vi "Periodic Tasks.vi"(8 "error in":errorcluster) -> ()   [LabVIEW 2016]
doc: "This VI runs in parallel to other tasks. It can contain as many user-defined periodic loops as you need. These can carry out PID or other sorts of timed response."
uses:
  <vilib>/Rock Robotics/WPI/DriverStation/WPI_DriverStationRobotMode2.ctl
  <vilib>/Rock Robotics/WPI/Utilities/WPI_GetSetVariantRefNum.vi
  Robot Global Data.vi
  <vilib>/Rock Robotics/WPI/RobotDrive/WPI_RobotDriveArcadeDrive_Standard(NoSaturation).vi
  <vilib>/Rock Robotics/Network Tables/NT Read String.vi
  <vilib>/Rock Robotics/Network Tables/NT Read Number.vi
  Drive Base Class/DriveBase.lvclass
panel:
  in  "Angle PID gains":T1
  out "Robot Mode":T2
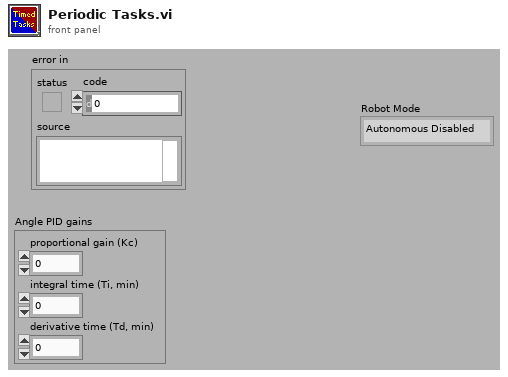
[diagram p1: front panel]
types:
  T1 = cluster{"proportional gain (Kc)":dbl, "integral time (Ti, min)":dbl, "derivative time (Td, min)":dbl}
  T2 = typedef "WPI_DriverStationRobotMode2.ctl" = enum16{"Autonomous Disabled", "Autonomous Enabled", "Teleop Disabled", "Teleop Enabled", "Disconnected", "Finish", "Test Disabled", "Test Enabled", "Emergency Stopped"}
  T3 = typedef "WPI_GyroDevRef.ctl" = cluster{"DevStatus":errorcluster, "Analog Channel":T4, "Offset":dbl, "Gain (VoltsPerDegree/Second)":dbl, "Gyro Type":enum16{"Analog", "XRS450"}, "Handle":i32, "SPI Bus":T5, "Device Found":bool, "Sample Rate":dbl, "Calibrate On Open":bool}
  T4 = typedef "FPGA_AIChannel.ctl" = enum8{"AI 0", "AI 1", "AI 2", "AI 3", "AI MXP 0", "AI MXP 1", "AI MXP 2", "AI MXP 3", "Invalid"}
  T5 = typedef "spi_bus.ctl" = enum16{"SPI On-Board, CS0", "SPI On-Board, CS1", "SPI On-Board, CS2", "SPI On-Board, CS3", "SPI MXP", "Invalid"}
  T6 = typedef "WPI_PotentiometerDevRef.ctl" = cluster{"DevStatus":errorcluster, "Analog Channel":T4, "Invert Output":bool}
  T7 = typedef "WPI_EncoderDevRef.ctl" = cluster{"DevStatus":errorcluster, "EncoderIndex":T8, "CounterIndex":T9, "DistancePerCount":dbl, "Decoding Type":T10}
  T8 = typedef "FPGA_EncoderIdx.ctl" = enum8{"Enc 0", "Enc 1", "Enc 2", "Enc 3", "Enc 4", "Enc 5", "Enc 6", "Enc 7", "Invalid"}
  T9 = typedef "FPGA_CounterCtrSystemIndex.ctl" = enum8{"Ctr 0", "Ctr 1", "Ctr 2", "Ctr 3", "Ctr 4", "Ctr 5", "Ctr 6", "Ctr 7", "Invalid"}
  T10 = typedef "WPI_EncoderType.ctl" = enum16{"1x", "2x", "4x"}
  T11 = cluster{"Right Encoder Distance":dbl, "Left Encoder Distance":dbl, "Right Encoder Velocity":dbl, "Left Encoder Velocity":dbl}
  T12 = cluster{"Yaw":dbl, "Roll":dbl, "Pitch":dbl, "Heading":dbl, "Fused Heading":dbl}
  T13 = typedef "WPI_RobotDriveDevRef.ctl" = cluster{"DevStatus":errorcluster, "Motors[]":T14[], "Square Inputs":bool, "Max Output":dbl}
  T14 = typedef "WPI_MotorControlDeviceRef.ctl" = cluster{"DeviceStatus":errorcluster, "Type":T15, "PWM":cluster{"PWM Channel":T16, "DeadBand":T17}, "CAN":cluster{"Device Number":u8, "SetOutput VI Ref":variant, "GetOutput VI Ref":variant, "Enable VI Ref":variant, "Disable VI Ref":variant, "Data":variant}, "Invert":bool}
  T15 = typedef "WPI_MotorControlType.ctl" = enum16{"PWM", "CAN"}
  T16 = typedef "FPGA_DIOPWMChannel.ctl" = enum8{"PWM 0", "PWM 1", "PWM 2", "PWM 3", "PWM 4", "PWM 5", "PWM 6", "PWM 7", "PWM 8", "PWM 9", "PWM MXP 0", "PWM MXP 1", "PWM MXP 2", "PWM MXP 3", "PWM MXP 4", "PWM MXP 5", "PWM MXP 6", "PWM MXP 7", "PWM MXP 8", "PWM MXP 9", "Invalid"}
  T17 = typedef "WPI_PWMDeadband.ctl" = cluster{"Name":string, "maxPositivePwm":i32, "minPositivePwm":i32, "centerPwm":i32, "maxNegativePwm":i32, "minNegativePwm":i32, "angularRange":u16}
  T18 = typedef "DriveBase.lvclass/DriveStates.ctl" = enum16{"Tank", "Arcade", "DriveStraight"}
  T19 = enum16{"open", "replace", "create", "open or create", "replace or create", "replace or create with confirmation"}
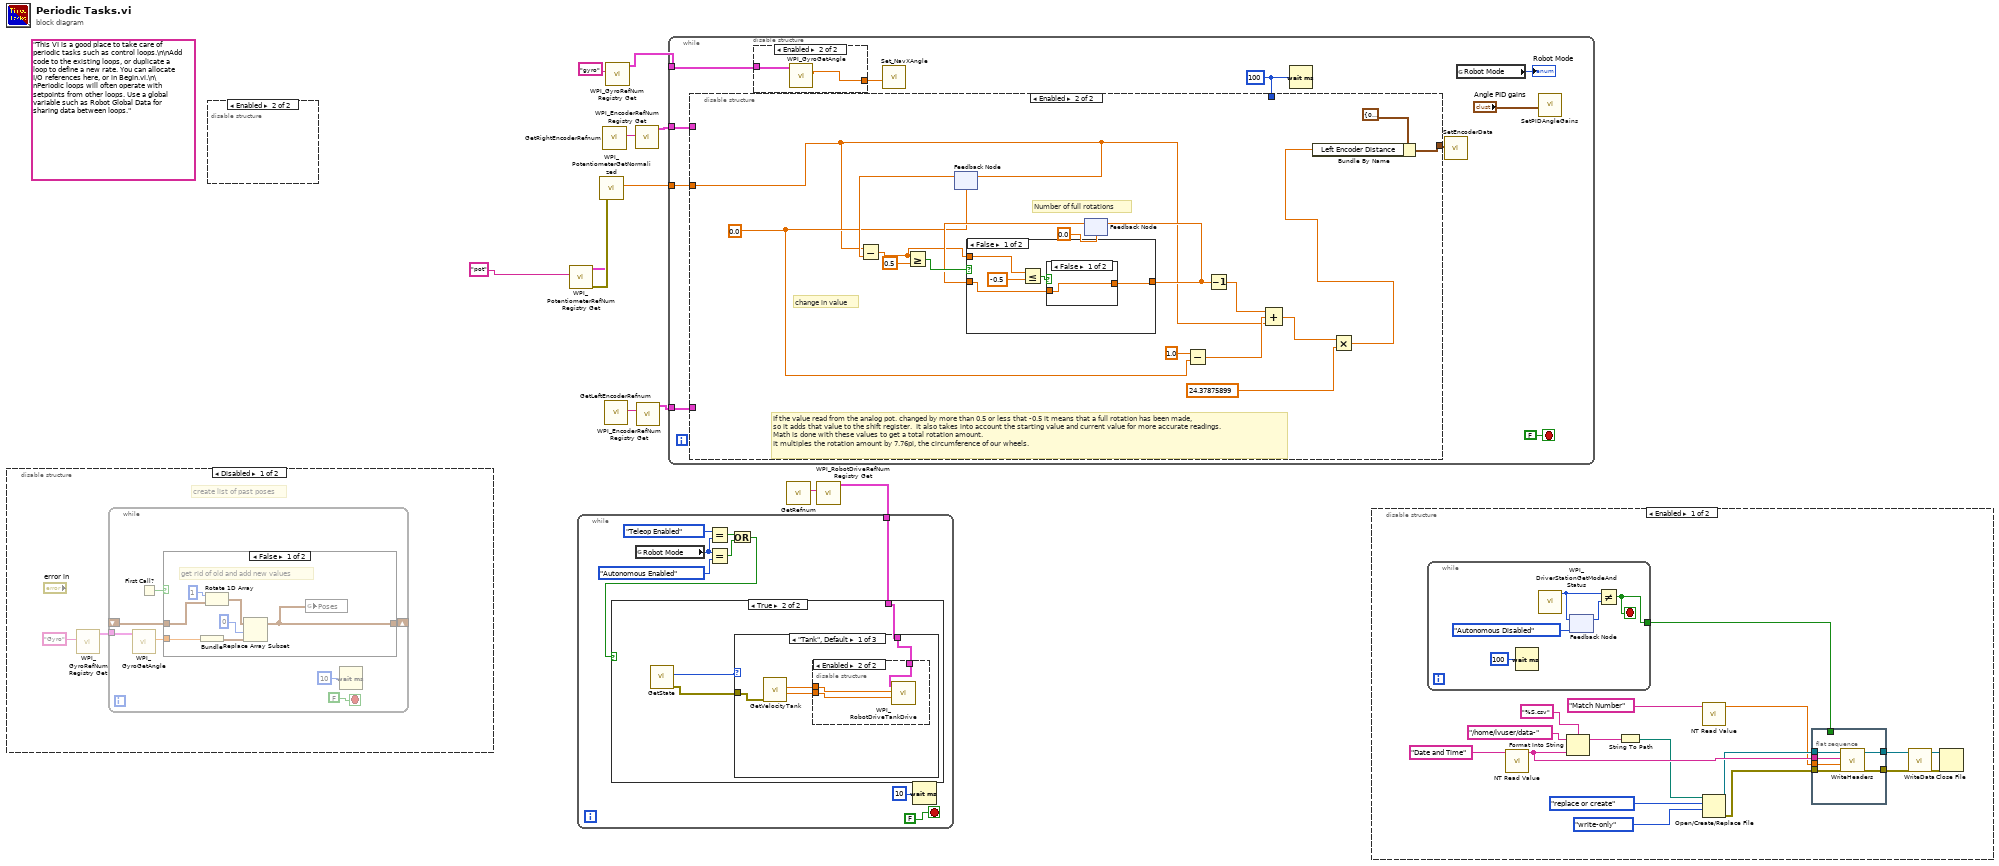
[diagram p0: block diagram]
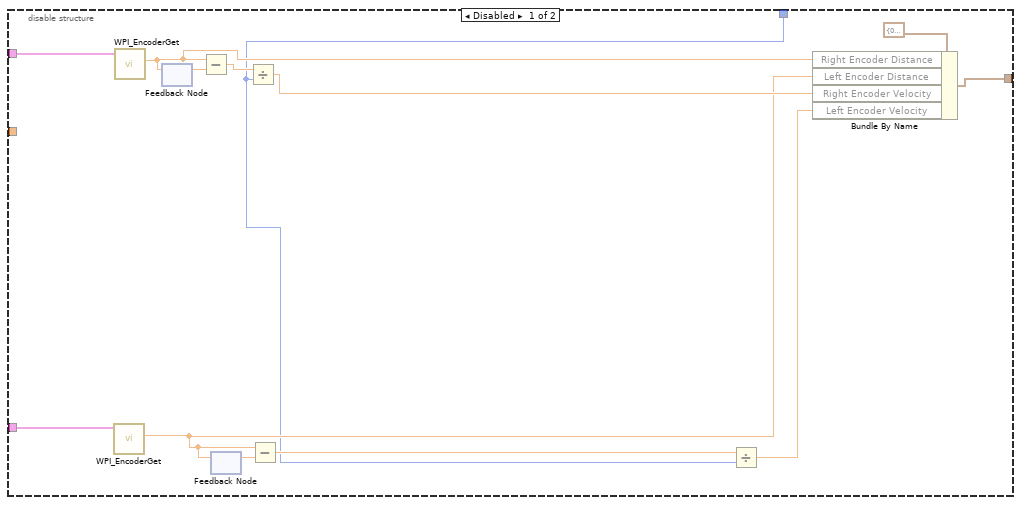
[diagram p2: hidden frame]
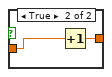
[diagram p3: hidden frame]
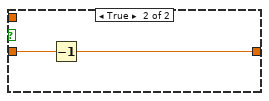
[diagram p4: hidden frame]
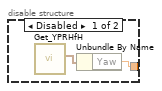
[diagram p5: hidden frame]
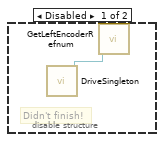
[diagram p7: hidden frame]
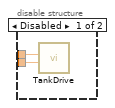
[diagram p9: hidden frame]
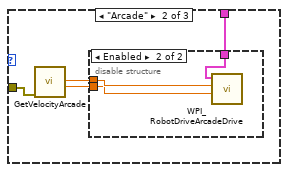
[diagram p10: hidden frame]
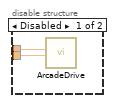
[diagram p11: hidden frame]
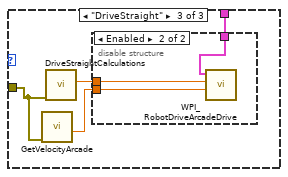
[diagram p12: hidden frame]
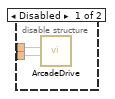
[diagram p13: hidden frame]
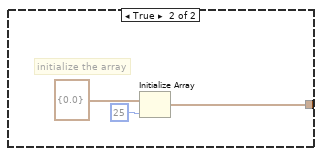
[diagram p14: hidden frame]
diagram:
  (unwired) "This VI is a good place to take care of periodic tasks such as control loops.\n\nAdd code to the existing loops, or duplicate a loop to define a new rate. You can allocate I/O references here, or in Begin.vi.\n\nPeriodic loops will often operate with setpoints from other loops. Use a global variable such as Robot Global Data for sharing data between loops."
  n1 = disable-structure shown="Disabled" {
    frame Disabled {
      # "create list of past poses"
      n2 = call <vilib>:"WPI_GyroRefNum Registry Get.vi"("refnum name"="Gyro") -> ("GyroDevRef"=w13:T3)  [unwired: 9 in, 1 out]
      n3 = while {
        tunnel: w13 -> [w19]
        shift-right: [w17] -> _
        shift-left: _ -> [w16]
        stop <- FALSE stop-if-true
        n4 = call <vilib>:"WPI_GyroGetAngle.vi"("GyroDevRef"=w19) -> ("Angle"=w15:dbl)  [unwired: 6 in, 4 out]
        n5 = First Call?() -> (First Call?: T/F=w18:bool)
        n6 = case shown="False" w18 {
          tunnel: [w22 w30] -> w17
          tunnel: w16 -> [w28 _]
          tunnel: w15 -> [w24 _]
          frame False {
            # "get rid of old and add new values"
            n7 = Bundle("Angle"=w24) -> (w23:cluster{"Angle":dbl})  [unwired: 1 in]
            n8 = Rotate 1D Array(1:w28, 2:1 ("n")) -> (0:w26:cluster{"theta":dbl}[])
            n9 = Replace Array Subset(array=w26, new element=w23, index=0) -> (w22:cluster{"theta":dbl}[])
            n10 = global write "Robot Global Data.vi" "Poses"(w22) -> ()
          }
          frame True {
            # "initialize the array"
            n11 = Initialize Array(cluster{"theta":dbl} {"theta"=0.0}, 25 ("dimension size")) -> (w30:cluster{"theta":dbl}[])
          }
        }
        n12 = Wait (ms)(milliseconds to wait=u32 10) -> ()  [unwired: 1 out]
      }
    }
    frame Enabled {
    }
  }
  n13 = disable-structure shown="Enabled" {
    frame Disabled {
      # "Didn't finish!"
      n14 = call "DriveSingleton.vi"() -> ("DriveBase.lvclass 2"=w32:refnum<class "DriveBase.lvclass">)  [unwired: 10 in, 1 out]
      n15 = call "GetLeftEncoderRefnum.vi"(11:w32) -> ()  [unwired: 10 in, 1 out]
    }
    frame Enabled {
    }
  }
  n16 = call <vilib>:"WPI_PotentiometerRefNum Registry Get.vi"("refnum name"="pot") -> ("error out"=w3:errorcluster, "PotDevRef"=w2:T6)  [unwired: 9 in]
  n17 = call <vilib>:"WPI_PotentiometerGetNormalized.vi"("error in"=w3, "PotDevRef"=w2) -> ("Normalized Value"=w4:dbl)  [unwired: 7 in, 2 out]
  n18 = call "GetRightEncoderRefnum.vi"() -> ("RightEncoderRefnum"=w5:string)  [unwired: 11 in]
  n19 = call "GetLeftEncoderRefnum.vi"() -> ("LeftEncoderRefnum"=w6:string)  [unwired: 11 in]
  n20 = call <vilib>:"WPI_GyroRefNum Registry Get.vi"("refnum name"="gyro") -> ("GyroDevRef"=w9:T3)  [unwired: 9 in, 1 out]
  n21 = call <vilib>:"WPI_EncoderRefNum Registry Get.vi"("refnum name"=w5) -> ("EncoderDevRef"=w8:T7)  [unwired: 9 in, 1 out]
  n22 = call <vilib>:"WPI_EncoderRefNum Registry Get.vi"("refnum name"=w6) -> ("EncoderDevRef"=w7:T7)  [unwired: 9 in, 1 out]
  n23 = while {
    tunnel: w9 -> [w38]
    tunnel: w8 -> [w37]
    tunnel: w7 -> [w36]
    tunnel: w4 -> [w33]
    stop <- FALSE stop-if-true
    w34 = u32 100 ("milliseconds to wait")
    n24 = disable-structure shown="Enabled" {
      disable-tunnel: w37 -> [w55 _]
      disable-tunnel: w36 -> [w54 _]
      disable-tunnel: [w44 w58] -> w35
      disable-tunnel: w34 -> [w43 _]
      disable-tunnel: w33 -> [_ w60]
      frame Disabled {
        n25 = call <vilib>:"WPI_EncoderGet.vi"("EncoderDevRef"=w54) -> ("Distance"=w46:dbl)  [unwired: 5 in, 5 out]
        n26 = call <vilib>:"WPI_EncoderGet.vi"("EncoderDevRef"=w55) -> ("Distance"=w52:dbl)  [unwired: 5 in, 5 out]
        n27 = feedback #1() -> (w53:dbl)  [unwired: 1 in]
        n28 = feedback-in #1(w52) -> ()
        n29 = Subtract(x=w52, y=w53) -> (x-y=w50:dbl)
        n30 = feedback #2() -> (w48:dbl)  [unwired: 1 in]
        n31 = feedback-in #2(w46) -> ()
        n32 = Divide(x=w50, y=w43) -> (x/y=w49:dbl)
        n33 = Subtract(x=w46, y=w48) -> (x-y=w47:dbl)
        n34 = Divide(x=w47, y=w43) -> (x/y=w45:dbl)
        n35 = Bundle By Name(cluster=T11 {"Right Encoder Distance"=0.0, "Left Encoder Distance"=0.0, "Right Encoder Velocity"=0.0, "Left Encoder Velocity"=0.0} ("Encoder Data"), "Right Encoder Distance"=w52, "Left Encoder Distance"=w46, "Right Encoder Velocity"=w49, "Left Encoder Velocity"=w45) -> (w44:T11)
      }
      frame Enabled {
        w61 = 0.0 ("y")
        # "change in value"
        # "Number of full rotations"
        # "If the value read from the analog pot. changed by more than 0.5 or less that -0.5 it means that a full rotation has been made, \nso it adds that value to the shift register.  It also takes into account the starting value and current value for more accurate readings.\nMath is done with these values to get a total rotation amount.\nIt multiples the rotation amount by 7.76pi, the circumference of our wheels."
        n36 = feedback #3(w61) -> (w64:dbl)
        n37 = Subtract(x=w60, y=w64) -> (x-y=w69:dbl)
        n38 = Greater Or Equal?(x=w69, y=0.5) -> (x >= y?=w71:bool)
        n39 = feedback-in #3(w60) -> ()
        n40 = feedback #4(0.0) -> (w70:dbl)
        n41 = case shown="False" w71 {
          tunnel: [w73 w82] -> w67
          tunnel: w70 -> [w74 w81]
          tunnel: w69 -> [w77 _]
          frame False {
            n42 = Less Or Equal?(x=w77, y=-0.5) -> (x <= y?=w75:bool)
            n43 = case shown="False" w75 {
              tunnel: w74 -> [w78 w80]
              tunnel: [w78 w79] -> w73
              frame False {
              }
              frame True {
                n44 = Increment(x=w80) -> (x+1=w79:dbl)
              }
            }
          }
          frame True {
            n45 = Decrement(x=w81) -> (x-1=w82:dbl)
          }
        }
        n46 = feedback-in #4(w67) -> ()
        n47 = Subtract(x=1.0, y=w61) -> (x-y=w65:dbl)
        n48 = Decrement(x=w67) -> (x-1=w66:dbl)
        n49 = Compound Arithmetic op=ADD(w66, w65, w60) -> (w62:dbl)
        n50 = Multiply(x=w62, y=24.37875899) -> (x*y=w57:dbl)
        n51 = Bundle By Name(cluster=T11 {"Right Encoder Distance"=0.0, "Left Encoder Distance"=0.0, "Right Encoder Velocity"=0.0, "Left Encoder Velocity"=0.0} ("Encoder Data"), "Left Encoder Distance"=w57) -> (w58:T11)
      }
    }
    n52 = disable-structure shown="Enabled" {
      disable-tunnel: [w83 w85] -> w42
      disable-tunnel: w38 -> [_ w86]
      frame Disabled {
        n53 = call <userlib>:"Get_YPRHfH.vi"() -> ("YRPHfH"=w84:T12)  [unwired: 11 in]
        n54 = Unbundle By Name(w84) -> ("Yaw"=w83:dbl)
      }
      frame Enabled {
        n55 = call <vilib>:"WPI_GyroGetAngle.vi"("GyroDevRef"=w86) -> ("Angle"=w85:dbl)  [unwired: 6 in, 4 out]
      }
    }
    n56 = call "Set_NavXAngle.vi"("NavX Angle"=w42) -> ()  [unwired: 11 in]
    n57 = Wait (ms)(milliseconds to wait=w34) -> ()  [unwired: 1 out]
    n58 = call "SetEncoderData.vi"("Encoder Data"=w35) -> ()  [unwired: 10 in, 1 out]
    n59 = global read "Robot Global Data.vi" "Robot Mode"() -> (→"Robot Mode":T2)
    n60 = call "SetPIDAngleGains.vi"("Angle PID gains"="Angle PID gains") -> ()  [unwired: 10 in, 1 out]
  }
  n61 = call "GetRefnum.vi"() -> ("RobotDriveRefnum"=w12:string)  [unwired: 10 in, 1 out]
  n62 = call <vilib>:"WPI_RobotDriveRefNum Registry Get.vi"("refnum name"=w12) -> ("RobotDriveDevRef"=w11:T13)  [unwired: 9 in, 1 out]
  n63 = while {
    tunnel: w11 -> [w93]
    stop <- FALSE stop-if-true
    n64 = global read "Robot Global Data.vi" "Robot Mode"() -> (w88:T2)
    n65 = Equal?(x=WPI_DriverStationRobotMode2."Teleop Enabled" ("Robot Mode"), y=w88) -> (x = y?=w91:bool)
    n66 = Equal?(x=w88, y=WPI_DriverStationRobotMode2."Autonomous Enabled" ("Robot Mode")) -> (x = y?=w90:bool)
    n67 = Or(x=w91, y=w90) -> (x .or. y?=w87:bool)
    n68 = case shown="True" w87 {
      tunnel: w93 -> [_ w98]
      frame False {
      }
      frame True {
        n69 = call "GetState.vi"() -> ("error out"=w96:errorcluster, "State"=w97:T18)  [unwired: 10 in]
        n70 = case shown="\"Tank\", Default" w97 {
          tunnel: w98 -> [w100 w109 w119]
          tunnel: w96 -> [w99 w108 w118]
          frame "Tank", Default {
            n71 = call "GetVelocityTank.vi"("error in (no error)"=w99) -> ("rightVelocitySetpointOutput"=w101:dbl, "leftVelocitySetpointOutput"=w102:dbl)  [unwired: 8 in, 1 out]
            n72 = disable-structure shown="Enabled" {
              disable-tunnel: w102 -> [w104 w107]
              disable-tunnel: w101 -> [w103 w106]
              disable-tunnel: w100 -> [_ w105]
              frame Disabled {
                n73 = call "TankDrive.vi"("Right"=w103, "Left"=w104) -> ()  [unwired: 10 in]
              }
              frame Enabled {
                n74 = call <vilib>:"WPI_RobotDriveTankDrive.vi"("Right axis value"=w106, "Left axis value"=w107, "RobotDriveDevRef"=w105) -> ()  [unwired: 6 in, 3 out]
              }
            }
          }
          frame "Arcade" {
            n75 = call "GetVelocityArcade.vi"("error in (no error)"=w108) -> ("Y Axis"=w110:dbl, "X Axis"=w111:dbl)  [unwired: 8 in, 1 out]
            n76 = disable-structure shown="Enabled" {
              disable-tunnel: w111 -> [w113 w116]
              disable-tunnel: w110 -> [w112 w115]
              disable-tunnel: w109 -> [_ w117]
              frame Disabled {
                n77 = call "ArcadeDrive.vi"("y-axis"=w112, "x-axis"=w113) -> (11:w114)  [unwired: 9 in]
              }
              frame Enabled {
                n78 = call-poly <vilib>:"WPI_RobotDriveArcadeDrive.vi"("Y axis value"=w115, "X axis value"=w116, "RobotDriveDevRef"=w117) -> ()  [unwired: 6 in, 3 out]
              }
            }
          }
          frame "DriveStraight" {
            n79 = call "GetVelocityArcade.vi"("error in (no error)"=w118) -> ("Y Axis"=w121:dbl)  [unwired: 8 in, 2 out]
            n80 = call "DriveStraightCalculations.vi"("error in (no error)"=w118) -> ("PIDOutput"=w120:dbl)  [unwired: 9 in, 1 out]
            n81 = disable-structure shown="Enabled" {
              disable-tunnel: w121 -> [w123 w124]
              disable-tunnel: w120 -> [w122 w125]
              disable-tunnel: w119 -> [_ w126]
              frame Disabled {
                n82 = call "ArcadeDrive.vi"("y-axis"=w123, "x-axis"=w122) -> ()  [unwired: 10 in]
              }
              frame Enabled {
                n83 = call-poly <vilib>:"WPI_RobotDriveArcadeDrive.vi"("Y axis value"=w124, "X axis value"=w125, "RobotDriveDevRef"=w126) -> ()  [unwired: 6 in, 3 out]
              }
            }
          }
        }
      }
    }
    n84 = Wait (ms)(milliseconds to wait=u32 10) -> ()  [unwired: 1 out]
  }
  n85 = disable-structure shown="Enabled" {
    frame Enabled {
      n86 = while {
        tunnel: [w148] -> w143
        stop <- w148 stop-if-true
        n87 = Wait (ms)(milliseconds to wait=u32 100) -> ()  [unwired: 1 out]
        n88 = call <vilib>:"WPI_DriverStationGetModeAndStatus.vi"() -> ("Robot Mode"=w145:T2)  [unwired: 10 in, 1 out]
        n89 = feedback #5(WPI_DriverStationRobotMode2."Autonomous Disabled" ("Robot Mode")) -> (w147:T2)
        n90 = feedback-in #5(w145) -> ()
        n91 = Not Equal?(x=w145, y=w147) -> (x != y?=w148:bool)
      }
      n92 = call-poly <vilib>:"NT Read Value.vi"("Name"="Date and Time") -> ("String"=w142:string)  [unwired: 9 in, 1 out]
      n93 = Format Into String(format string="%S.csv", initial string="/home/lvuser/data-", w142) -> (resulting string=w140:string)  [unwired: 1 in, 1 out]
      n94 = String To Path(string=w140) -> (path=w137:path)
      n95 = call-poly <vilib>:"NT Read Value.vi"("Name"="Match Number") -> ("Numeric"=w132:dbl)  [unwired: 9 in, 1 out]
      n96 = Open/Create/Replace File(file path (use dialog)=w137, operation (0:open)=T19."replace or create", access (0:read/write)=enum16{"read/write", "read-only", "write-only"}."write-only") -> (refnum out=w135:refnum<file>, error out=w136:errorcluster)  [unwired: 3 in, 1 out]
      n97 = flat-sequence {
        tunnel: w142 -> [w154]
        tunnel: w132 -> [w149]
        tunnel: w135 -> [w150]
        tunnel: [w151] -> w130
        tunnel: [w152] -> w127
        tunnel: w136 -> [w153]
        tunnel: w143 -> [_]
        frame #0 {
          n98 = call "WriteHeaders.vi"("error in"=w153, "Match Number"=w149, "Date and Time"=w154, "File in"=w150) -> ("error out"=w152:errorcluster, "File out"=w151:refnum<file>)  [unwired: 6 in]
        }
      }
      n99 = call "WriteData.vi"("error in"=w127, "File in"=w130) -> ("error out"=w129:errorcluster, "refnum out"=w128:refnum<file>)  [unwired: 8 in]
      n100 = Close File(refnum=w128, error in=w129) -> ()  [unwired: 2 out]
    }
    frame Disabled {
    }
  }
